vi "Reset old test Values (SubVI).vi"(8 "error in":errorcluster, 9 "Atr in":refnum<vi>, 11 "Test Paragraph":string) -> (0 "error out":errorcluster)   [LabVIEW 2017]
uses:
  <vilib>/Utility/miscctls.llb/LVRowAndColumnTypeDef.ctl
panel:
  out "concatenated string":string
  out "Value":string[][](array[string])
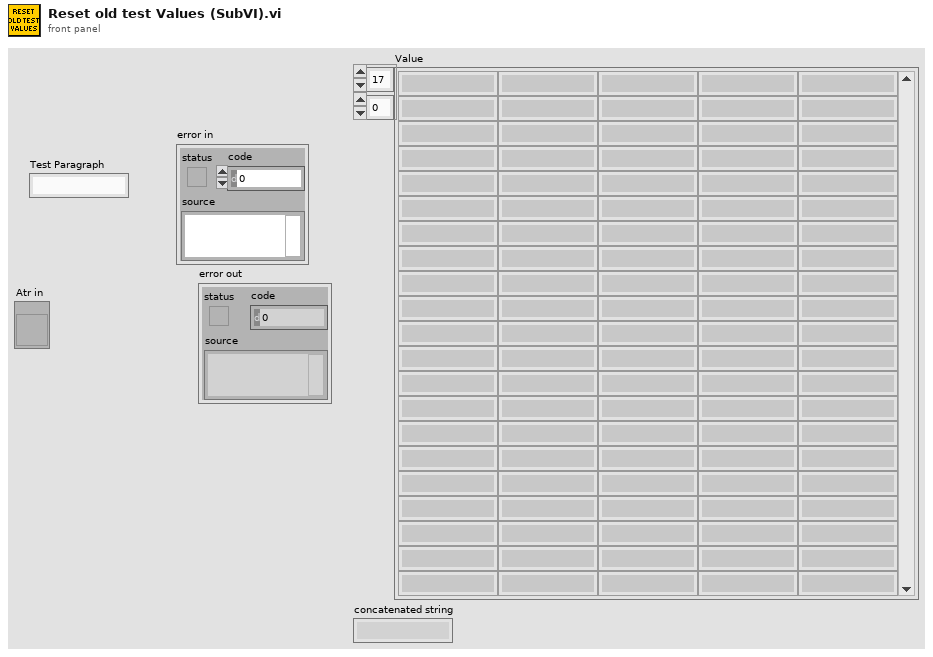
[diagram p1: front panel]
types:
  T1 = typedef "LVRowAndColumnTypeDef.ctl" = cluster{"Row":i32, "Column":i32}
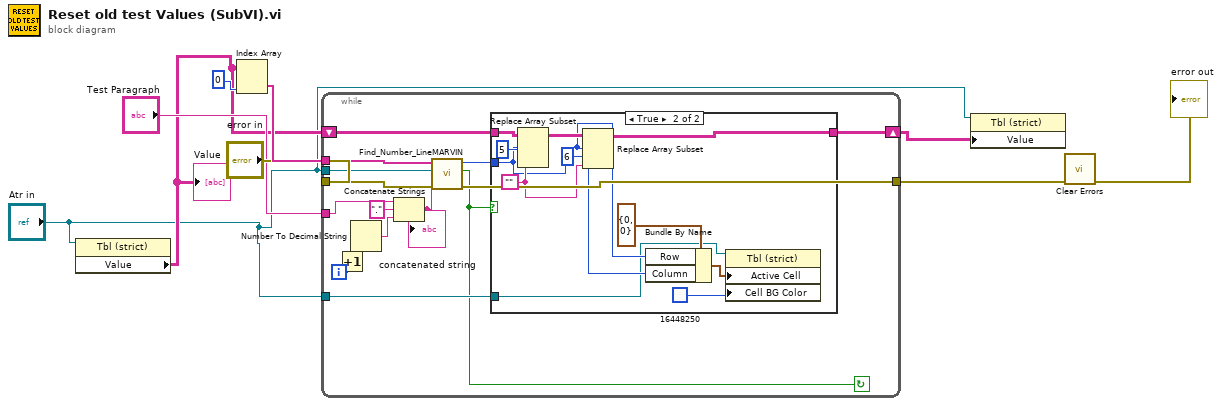
[diagram p0: block diagram]
diagram:
  n1 = property class="Tbl (strict)"(reference="Atr in") -> ("Value"=w4:string[][])  [unwired: 1 in, 2 out]
  "Value" <- w4
  n2 = Index Array(array=w4, index (col)=0 ("disabled index (col)")) -> (element=w8:string[])  [unwired: 1 in]
  n3 = while {
    tunnel: w8 -> [w24]
    tunnel: "Test Paragraph" -> [w21]
    tunnel: "error in" -> [w23]
    tunnel: [w22] -> w6
    shift-right: [w17] -> w2
    shift-left: w4 -> [w16]
    tunnel: "Atr in" -> [w13]
    tunnel: "Atr in" -> [w10]
    i -> [w15]
    stop <- w12 continue-if-true
    n4 = Increment(x=w15) -> (x+1=w11:i32)
    n5 = Number To Decimal String(number=w11) -> (decimal integer string=w19:string)  [unwired: 1 in]
    n6 = Concatenate Strings(w21, "." ("string"), w19) -> (w18:string)
    "concatenated string" <- w18
    n7 = call "Find_Number_LineMARVIN.vi"("Test Paragraph"=w18, "error in"=w23, "TableIn"=w10, "Row Headers[]"=w24) -> ("error out"=w22:errorcluster, "Found"=w12:bool, "Line number"=w14:i32)  [unwired: 1 in, 1 out]
    n8 = case shown="True" w12 {
      tunnel: [w25 w35] -> w17
      tunnel: w16 -> [w25 w34]
      tunnel: w14 -> [_ w29]
      tunnel: w13 -> [_ w26]
      frame False {
      }
      frame True {
        w32 = ""
        w28 = 6 ("disabled index (col)")
        n9 = Replace Array Subset(array=w34, new element=w32, index (row)=w29, index (col)=5 ("disabled index (col)")) -> (w36:string[][])
        n10 = Replace Array Subset(array=w36, new element=w32, index (row)=w29, index (col)=w28) -> (w35:string[][])
        n11 = Bundle By Name(cluster=T1 {"Row"=0, "Column"=0} ("Active Cell:Active Cell"), "Row"=w29, "Column"=w28) -> (w31:T1)
        n12 = property class="Tbl (strict)"(reference=w26, "Active Cell"=w31, "Cell BG Color"=u32 16448250) -> ()  [unwired: 1 in, 2 out]
      }
    }
  }
  n13 = property class="Tbl (strict)"(reference="Atr in", "Value"=w2) -> ()  [unwired: 1 in, 2 out]
  n14 = call <vilib>:"Clear Errors.vi"("error in (no error)"=w6) -> ("error out"=→"error out":errorcluster)  [unwired: 5 in, 1 out]
